vi "High Winds.vi"(1 "Wind Speed":dbl) -> (0 "High Winds":bool)   [LabVIEW 2019]
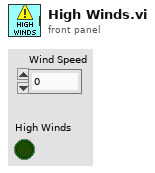
[diagram p1: front panel]
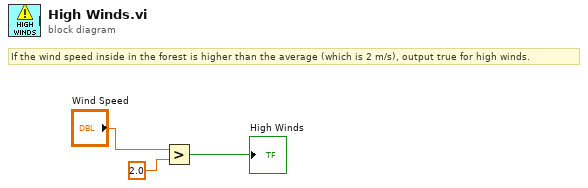
[diagram p0: block diagram]
diagram:
  # "If the wind speed inside in the forest is higher than the average (which is 2 m/s), output true for high winds."
  n1 = Greater?(x="Wind Speed", y=2.0) -> (0:→"High Winds":bool)
